vi "CountTimeouts.vi"(8 "Timed out":bool, 11 "Extra samples":i16) -> (0 "Valid sample":bool, 1 "Reset":bool, 2 "Extra sample":bool)   [LabVIEW 2013]
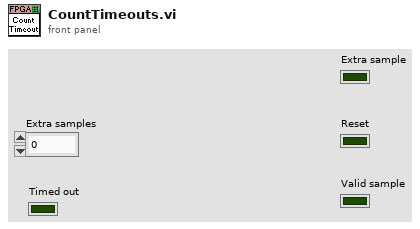
[diagram p1: front panel]
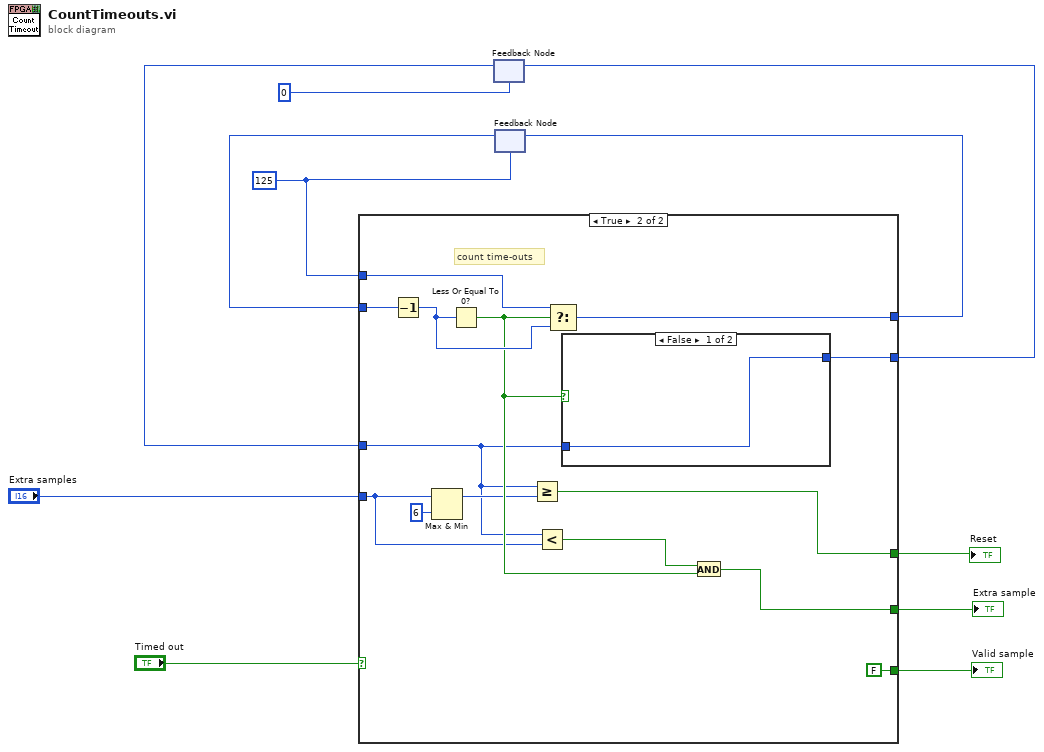
[diagram p0: block diagram]
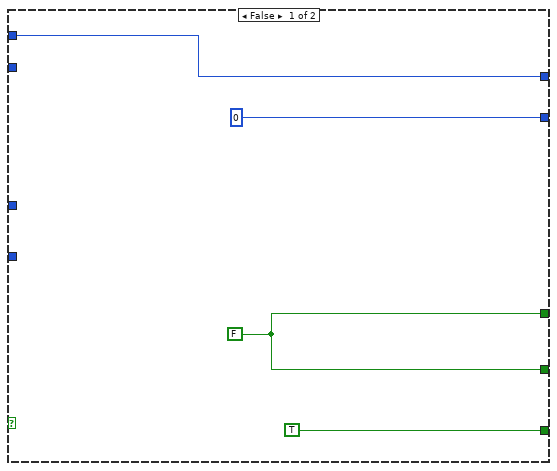
[diagram p2: hidden frame]
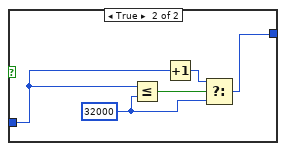
[diagram p3: hidden frame]
diagram:
  w9 = i16 125 ("Extra samples")
  n1 = feedback #1(i16 0 ("Extra samples")) -> (w1:i16)
  n2 = feedback #2(w9) -> (w10:i16)
  n3 = case shown="True" "Timed out" {
    tunnel: w10 -> [_ w29]
    tunnel: w9 -> [w15 w27]
    tunnel: [w15 w26] -> w8
    tunnel: [TRUE FALSE] -> w7
    tunnel: [w13 w23] -> w6
    tunnel: [w13 w22] -> w5
    tunnel: [i16 0 ("Extra samples") w24] -> w3
    tunnel: "Extra samples" -> [_ w17]
    tunnel: w1 -> [_ w18]
    frame False {
      w13 = FALSE
    }
    frame True {
      # "count time-outs"
      n4 = Decrement(x=w29) -> (x-1=w28:i16)
      n5 = Max & Min(x=w17, y=i16 6) -> (max(x,y)=w19:i16)  [unwired: 1 out]
      n6 = Less Or Equal To 0?(x=w28) -> (x <= 0?=w21:bool)
      n7 = Greater Or Equal?(x=w18, y=w19) -> (x >= y?=w23:bool)
      n8 = Less?(x=w18, y=w17) -> (x < y?=w16:bool)
      n9 = Select(t=w27, s=w21, f=w28) -> (s? t:f=w26:i16)
      n10 = case shown="False" w21 {
        tunnel: [w30 w33] -> w24
        tunnel: w18 -> [w30 w31]
        frame False {
        }
        frame True {
          w34 = i16 32000 ("y")
          n11 = Less Or Equal?(x=w31, y=w34) -> (x <= y?=w32:bool)
          n12 = Increment(x=w31) -> (x+1=w35:i16)
          n13 = Select(t=w35, s=w32, f=w34) -> (s? t:f=w33:i16)
        }
      }
      n14 = And(x=w16, y=w21) -> (x .and. y?=w22:bool)
    }
  }
  "Reset" <- w6
  "Valid sample" <- w7
  "Extra sample" <- w5
  n15 = feedback-in #1(w3) -> ()
  n16 = feedback-in #2(w8) -> ()
